vi "Peek or default.vi"(8 "error in (no error)":errorcluster, 10 "Default":bool=TRUE, 11 "Signaller in":refnum<class "Signaller.lvclass">) -> (0 "error out":errorcluster, 2 "Has signal?":bool, 3 "Signaller out":refnum<class "Signaller.lvclass">)   [LabVIEW 2019, in "Signaller.lvclass"]
uses:
  Signaller.lvclass
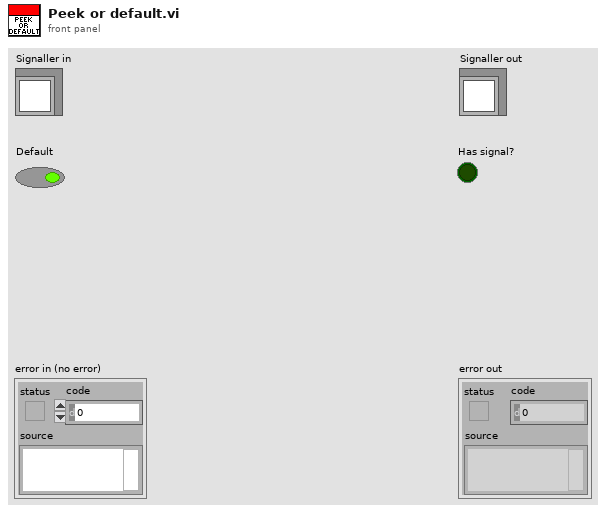
[diagram p1: front panel]
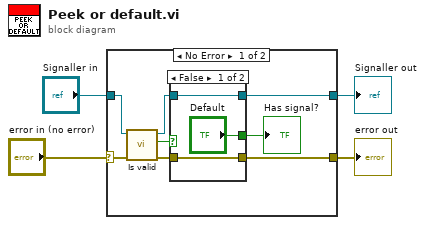
[diagram p0: block diagram]
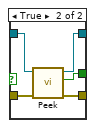
[diagram p2: hidden frame]
diagram:
  n1 = case shown="No Error" "error in (no error)" {
    selector: "error in (no error)" -> [w10 w22]
    tunnel: [w8 w22] -> w3
    tunnel: [w6 w21] -> w1
    tunnel: "Signaller in" -> [w11 w21]
    frame No Error {
      n2 = call "Is valid.vi"("error in (no error)"=w10, "Signaller in"=w11) -> ("error out"=w9:errorcluster, "Is valid?"=w12:bool, "Signaller out"=w7:refnum<class "Signaller.lvclass">)  [unwired: 7 in]
      n3 = case shown="False" w12 {
        tunnel: w9 -> [w13 w20]
        tunnel: [w13 w19] -> w8
        tunnel: w7 -> [w15 w18]
        tunnel: [w15 w17] -> w6
        tunnel: ["Default" w16] -> w5
        frame False {
        }
        frame True {
          n4 = call "Peek.vi"("error in (no error)"=w20, "Signaller in"=w18) -> ("error out"=w19:errorcluster, "Has signal"=w16:bool, "Signaller out"=w17:refnum<class "Signaller.lvclass">)  [unwired: 7 in]
        }
      }
      "Has signal?" <- w5
    }
    frame Error {
    }
  }
  "error out" <- w3
  "Signaller out" <- w1
